vi "HIOKI PW3390 CLS.vi"(6 "OPC query (T: ON)":bool=TRUE, 8 "error in (no error)":errorcluster, 11 "VISA Resource":refnum<visa-resource-name>) -> (0 "error out":errorcluster, 3 "VISA Resource out":refnum<visa-resource-name>)   [LabVIEW 2009]
doc: "Clears the event register."
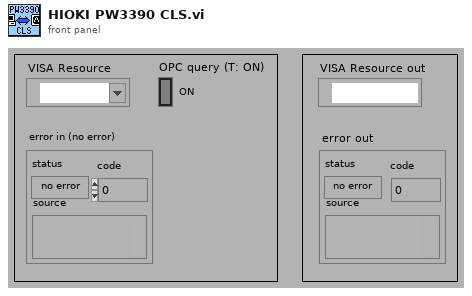
[diagram p1: front panel]
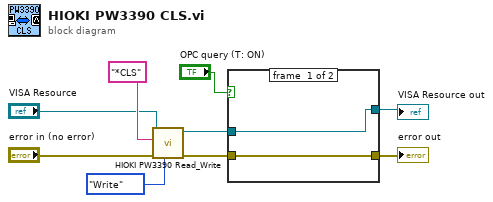
[diagram p0: block diagram]
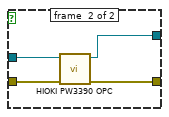
[diagram p2: hidden frame]
diagram:
  n1 = call <instrlib>:"HIOKI PW3390 Read_Write.vi"("Read/Write"=enum16{"Read", "Write"}."Write", "error in (no error)"="error in (no error)", "data in"="*CLS", "VISA Resource"="VISA Resource") -> ("error out"=w1:errorcluster, "VISA Resource out"=w4:refnum<visa-resource-name>)  [unwired: 5 in, 1 out]
  n2 = case shown="TRUE" "OPC query (T: ON)" {
    tunnel: w4 -> [w11 w15]
    tunnel: [w11 w14] -> w3
    tunnel: [w10 w13] -> w2
    tunnel: w1 -> [w10 w12]
    frame #0 {
    }
    frame #1 {
      n3 = call <instrlib>:"HIOKI PW3390 OPC.vi"("error in (no error)"=w12, "VISA Resource"=w15) -> ("error out"=w13:errorcluster, "VISA Resource out"=w14:refnum<visa-resource-name>)  [unwired: 7 in, 1 out]
    }
  }
  "error out" <- w2
  "VISA Resource out" <- w3
